vi "Control - Generic - High-Idle Governor Host.vi"() -> ()   [LabVIEW 2015, in "ECS-Host.lvlib"]
uses:
  ECS-Host.lvlib
panel:
  out "PedalOut":sgl caption="[]"
  out "PedalIn":sgl caption="[%]"
  out "HIG_DEffort":sgl caption="[]"
  out "HIG_IEffort":sgl caption="[]"
  out "HIG_PEffort":sgl caption="[]"
  in  "HIG_IntMin":sgl caption="[]"
  in  "HIG_IntMax":sgl caption="[]"
  in  "HIG_DerMin":sgl caption="[]"
  in  "HIG_DerMax":sgl caption="[]"
  out "HIG_PIDOut":sgl caption="[]"
  in  "HIG_Kd":sgl caption="[]"
  in  "HIG_PIDMin":sgl caption="[]"
  in  "HIG_PIDMax":sgl caption="[]"
  in  "HIG_Ki":sgl caption="[%-sec/RPM]"
  in  "HIG_Kp":sgl caption="[%/RPM]"
  in  "HighIdleSpeed":sgl caption="[RPM]"
  in  "HIG_E":bool
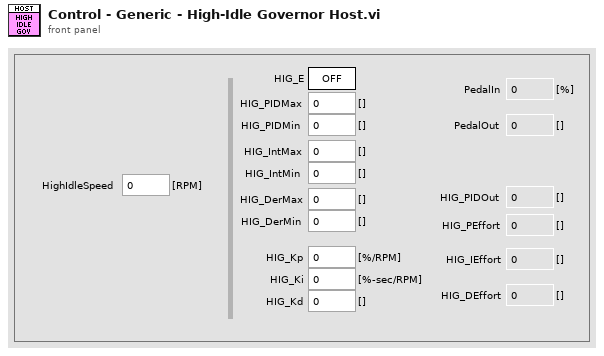
[diagram p1: front panel]
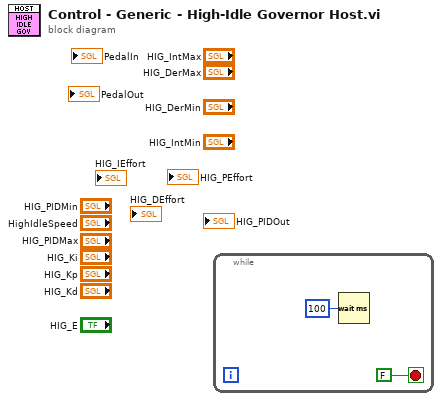
[diagram p0: block diagram]
diagram:
  n1 = while {
    stop <- FALSE stop-if-true
    n2 = Wait (ms)(milliseconds to wait=u32 100) -> ()  [unwired: 1 out]
  }
